vi "LVClasse_SurfaceFloat Get Data.vi"(0 "SurfaceFloat in":refnum<class "SurfaceFloat.lvclass">, 11 "error in (no error)":errorcluster) -> (4 "SurfaceFloat out":refnum<class "SurfaceFloat.lvclass">, 6 "data":sgl[][](array[numeric]), 15 "error out":errorcluster)   [LabVIEW 2020, in "SurfaceFloat.lvclass"]
doc: "Get read access Surface buffer.\n\n--------------------------------------------------------------------------------\n\n<B>SurfaceIn </B> : Surface object.\n<B>SurfaceOut </B> : Surface object.\n<B>data </B> : Surface buffer.\n<B>ErrorIn </B> : Error\n<B>ErrorOut </B> : Error\n\n--------------------------------------------------------------------------------"
uses:
  SurfaceFloat.lvclass
  SurfaceFloat.lvclass/SurfaceFloat.ctl
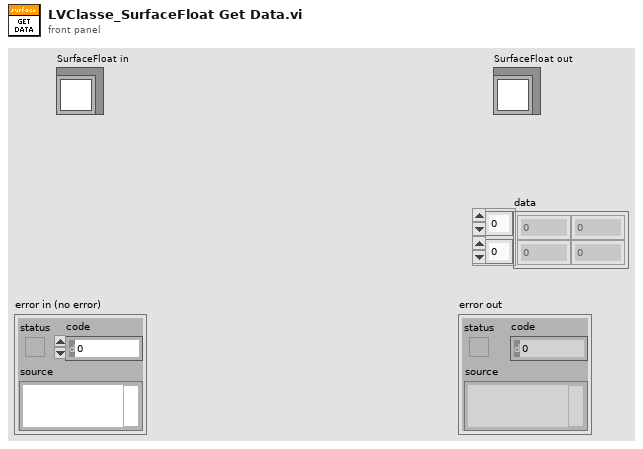
[diagram p1: front panel]
types:
  T1 = typedef "General dimensions definition.ctl" = cluster{"Size":T2, "Step":T3}
  T2 = typedef "Point2D.ctl" = cluster{"X":u32, "Y":u32}
  T3 = typedef "Point2Df.ctl" = cluster{"X":sgl, "Y":sgl}
  T4 = typedef "ClassID.ctl" = i64
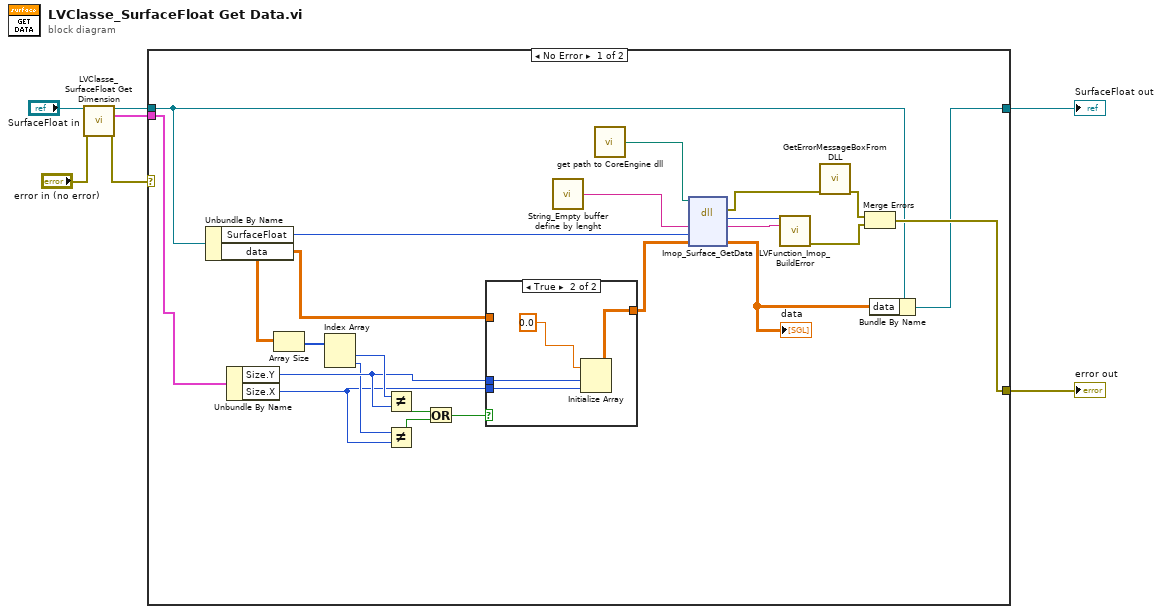
[diagram p0: block diagram]
diagram:
  n1 = call "LVClasse_SurfaceFloat Get Dimension.vi"("SurfaceFloat in"="SurfaceFloat in", "error in (no error)"="error in (no error)") -> ("SurfaceFloat out"=w4:refnum<class "SurfaceFloat.lvclass">, "Dimensions_um"=w1:T1, "error out"=w2:errorcluster)  [unwired: 11 in]
  n2 = case shown="No Error" w2 {
    selector: w2 -> [_ w37]
    tunnel: [w22 w37] -> w7
    tunnel: [w9 w36] -> w6
    tunnel: w4 -> [w10 w36]
    tunnel: w1 -> [w13 _]
    frame No Error {
      n3 = Unbundle By Name(w10) -> ("SurfaceFloat"=w25:T4, "data"=w11:sgl[][])
      n4 = Unbundle By Name(w13) -> ("Size.Y"=w19:u32, "Size.X"=w17:u32)
      n5 = Array Size(array=w11) -> (size(s)=w21:i32[])
      n6 = Index Array(array=w21) -> (element #1=w20:i32, element #2=w18:i32)  [unwired: 2 in]
      n7 = Not Equal?(x=w20, y=w19) -> (x != y?=w16:bool)
      n8 = Not Equal?(x=w18, y=w17) -> (x != y?=w15:bool)
      n9 = Or(x=w16, y=w15) -> (x .or. y?=w14:bool)
      n10 = case shown="True" w14 {
        tunnel: [w31 w33] -> w12
        tunnel: w19 -> [_ w35]
        tunnel: w17 -> [_ w34]
        tunnel: w11 -> [w31 _]
        frame False {
        }
        frame True {
          n11 = Initialize Array(sgl 0.0, w35, w34) -> (w33:sgl[][])
        }
      }
      n12 = call "String_Empty buffer define by lenght.vi"() -> ("Empty buffer"=w28:string)  [unwired: 1 in]
      n13 = call "get path to CoreEngine dll.vi"() -> ("path to wavekit library"=w27:path)  [unwired: 14 in, 1 out]
      n14 = dll-call lib="D:/2_trunk/Soft_haso/ImOpCoreEngine4_LV2011/DLLs/ImopEngine4_vc100.dll" fn="Imop_Surface_GetData"(path in=w27, "message"=w28, "surface"=w25, "data"=w12) -> (error out=w26:errorcluster, "return type"=w30:i32, "message"=w29:string, "data"=w8:sgl[][])  [unwired: 3 in, 1 out]
      "data" <- w8
      n15 = call "LVFunction_Imop_BuildError.vi"("code"=w30, "String to Prepend to source (\"\")"=w29) -> ("error out"=w23:errorcluster)  [unwired: 13 in]
      n16 = call "GetErrorMessageBoxFromDLL.vi"("error IN"=w26) -> ("error OUT"=w24:errorcluster)  [unwired: 10 in]
      n17 = Merge Errors(w24, w23) -> (w22:errorcluster)
      n18 = Bundle By Name(cluster=w10, "data"=w8) -> (w9:refnum<class "SurfaceFloat.lvclass">)
    }
    frame Error {
    }
  }
  "error out" <- w7
  "SurfaceFloat out" <- w6
